vi "CANopenVM_57_single.vi"(0 "node-ID":u8=1 min=1 max=127 step=1, 1 "目标速度":i16=50) -> (2 "电机绝对位置":i32=443333152, 3 "速度反馈值":i32=300, 4 "转矩反馈值 0.1%":i16=40)   [LabVIEW 2020]
uses:
  <vilib>/Platform/TimedLoop/XDataNode/timing_clust.ctl
  <vilib>/Platform/TimedLoop/XDataNode/nitl_modes.ctl
  <vilib>/Platform/TimedLoop/XDataNode/wakeup.ctl
  <vilib>/CANopenLib/CANOPEN.llb/CANopen Interface Create.vi
  <vilib>/CANopenLib/CANOPEN.llb/CANopen SDO Create.vi
  <vilib>/CANopenLib/CANOPEN.llb/CANopen SDO Write [I16].vi
  <vilib>/CANopenLib/CANOPEN.llb/CANopen SDO Close.vi
  <vilib>/CANopenLib/CANOPEN.llb/CANopen SYNC Create.vi
  <vilib>/CANopenLib/CANOPEN.llb/CANopen RPDO Create.vi
  <vilib>/CANopenLib/CANOPEN.llb/CANopen TPDO Create.vi
  <vilib>/CANopenLib/CANOPEN.llb/CANopen TPDO Start.vi
  <vilib>/CANopenLib/CANOPEN.llb/CANopen SYNC Start.vi
  <vilib>/CANopenLib/CANOPEN.llb/CANopen RPDO Start.vi
  <vilib>/CANopenLib/CANOPEN.llb/CANopen Convert To Data [I16].vi
  <vilib>/CANopenLib/CANOPEN.llb/CANopen Fetch from Data [I16].vi
  <vilib>/CANopenLib/CANOPEN.llb/CANopen Fetch from Data [I32].vi
  <vilib>/CANopenLib/CANOPEN.llb/CANopen SYNC Close.vi
  <vilib>/CANopenLib/CANOPEN.llb/CANopen RPDO Close.vi
  <vilib>/CANopenLib/CANOPEN.llb/CANopen TPDO Close.vi
  <vilib>/CANopenLib/CANOPEN.llb/CANopen Interface Close.vi
  <vilib>/Platform/TimedLoop/XDataNode/XDataNode.xnode
  <vilib>/Platform/TimedLoop/XDataNode/XDNodeRunTimeDep.lvlib
panel:
  out "completion code 4":u32
  out "completion code 3":u32
  out "completion code":u32
  in  "buffer size (0) 2":u16
  in  "TPDO channel":u8(ring)=2 items=["PDO 1", "PDO 2", "PDO 3", "PDO 4"]
  in  "Set Target Vilocity":i16
  in  "stop":bool
  out "timestamp":timestamp=timestamp(3824613290.037175 s since 1904-01-01)
  in  "buffer size (0)":u16=10
  in  "TPDO channel read":u8(ring)=1 items=["PDO 1", "PDO 2", "PDO 3", "PDO 4"]
  in  "RPDO channel write":u8(ring)=1 items=["PDO 1", "PDO 2", "PDO 3", "PDO 4"]
  in  "period (ms)":i64=10
  out "completion code 2":u32
  out "completion code 1":u32
  in  "batch SDO name":string="NiMotion_VM"
  in  "baud rate":u32(ring) items=["1 Mbit/s"=0, "800 kbit/s"=1, "500 kbit/s"=2, "250 kbit/s"=3, "125 kbit/s"=4, "50 kbit/s"=6, "20 kbit/s"=7, "10 kbit/s"=8]
  in  "CANopen interface":u32(ring) items=["CANopen01", "CANopen02", "CANopen03", "CANopen04", "CANopen05", "CANopen06", "CANopen07", "CANopen08", "CANopen09", "CANopen10", "CANopen11", "CANopen12", "CANopen13", "CANopen14", "CANopen15", "CANopen16", "CANopen17", "CANopen18", "CANopen19", "CANopen20", "CANopen21", "CANopen22", "CANopen23", "CANopen24", "CANopen25", "CANopen26", "CANopen27", "CANopen28", "CANopen29", "CANopen30", "CANopen31", "CANopen32"]
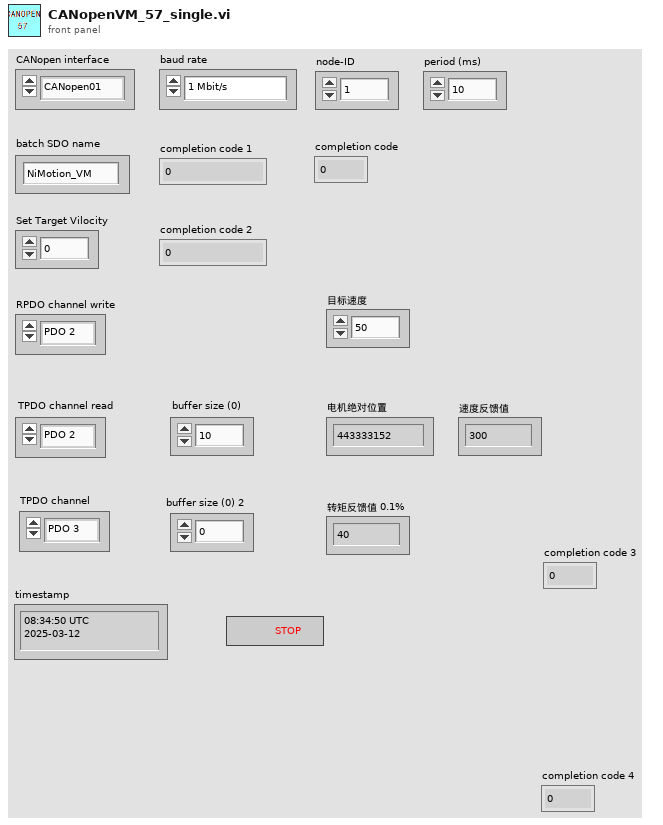
[diagram p1: front panel]
types:
  T1 = typedef "XDNodeRunTimeDep.lvlib/timing_clust.ctl" = cluster{"Expected End [f-1]":u64, "Actual End [f-1]":u64, "Finished Late? [f-1]":bool, "Expected End [i-1]":u64, "Actual End [i-1]":u64, "Finished Late? [i-1]":bool, "Expected Start [i]":u64, "Actual Start [i]":u64, "Expected Start [f]":u64, "Actual Start [f]":u64, "Source Name":string, "Structure Name":string, "Period":i64, "Deadline":i64, "Offset":i64, "Start":i64, "Priority":i32, "Timeout":i32, "Mode":T2, "Wakeup Reason":T3, "Error":errorcluster, "Source Type":string, "Secondary Source Type":string, "Global End Time":u64, "Global Start Time":u64, "Frame Duration":u64, "Iteration Duration":u64, "Assigned CPU":i32, "I/O Scan Engine Mode":u32}
  T2 = typedef "XDNodeRunTimeDep.lvlib/nitl_modes.ctl" = enum32{"No Change", "Process missed periods, maintain original phase", "Discard missed periods, maintain original phase", "Process missed periods, ignore original phase", "Discard missed periods, ignore original phase"}
  T3 = typedef "XDNodeRunTimeDep.lvlib/wakeup.ctl" = enum32{"Normal", "Aborted", "Asynchronous wakeup", "Timing source error", "Timed loop error", "Timeout"}
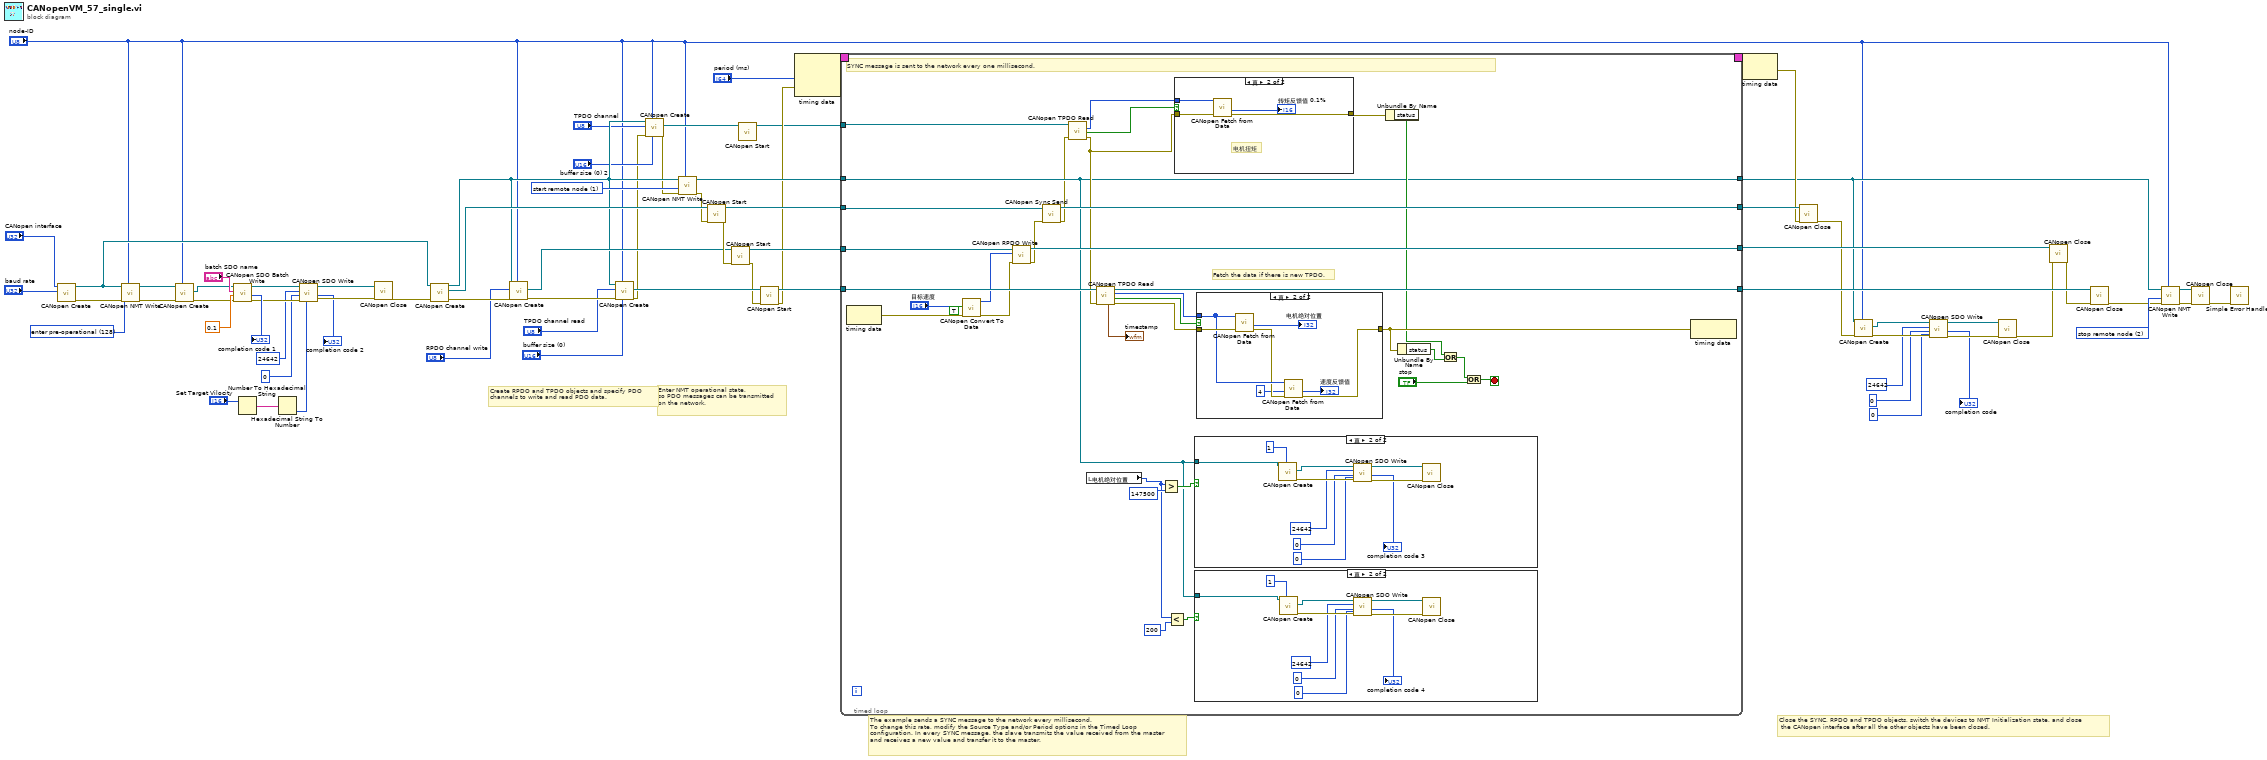
[diagram p0: block diagram]
diagram:
  w37 = u16 2 items=["start remote node"=1, "stop remote node"=2, "enter pre-operational"=128, "reset node"=129, "reset communication"=130] ("command")
  w49 = u16 1 items=["start remote node"=1, "stop remote node"=2, "enter pre-operational"=128, "reset node"=129, "reset communication"=130] ("command")
  w65 = u16 128 items=["start remote node"=1, "stop remote node"=2, "enter pre-operational"=128, "reset node"=129, "reset communication"=130] ("command")
  # "SYNC message is sent to the network every one millisecond."
  # "Close the SYNC, RPDO and TPDO objects, switch the devices to NMT Initialization state, and close\n the CANopen interface after all the other objects have been closed."
  # "The example sends a SYNC message to the network every millisecond.\nTo change this rate, modify the Source Type and/or Period options in the Timed Loop\nconfiguration. In every SYNC message, the slave transmits the value received from the master\nand receives a new value and transfer it to the master."
  # "Enter NMT operational state,\nso PDO messages can be transmitted\non the network."
  # "Create RPDO and TPDO objects and specify PDO \nchannels to write and read PDO data."
  n1 = call-poly <vilib>:"CANopen Create.vi"("baud rate"="baud rate", "interface name"="CANopen interface") -> ("error out"=w66:errorcluster, "interface object out"=w41:refnum<k20>)  [unwired: 8 in]
  n2 = call <vilib>:"CANopen NMT Write.vi"("node-ID (0)"="node-ID", "error in (no error)"=w66, "command"=w65, "interface object in"=w41) -> ("error out"=w69:errorcluster, "interface object out"=w70:refnum<k20>)  [unwired: 6 in]
  n3 = call-poly <vilib>:"CANopen Create.vi"("node-ID"="node-ID", "error in (no error)"=w69, "interface object in"=w70) -> ("error out"=w56:errorcluster, "SDO object out"=w62:refnum<k20>)  [unwired: 6 in, 1 out]
  n4 = call <vilib>:"CANopen SDO Batch Write.vi"("error in (no error)"=w56, "timeout (1s)"=0.1 ("timeout (0s)"), "batch SDO name"="batch SDO name", "SDO object in"=w62) -> ("error out"=w57:errorcluster, "completion code"=→"completion code 1":u32, "SDO object out"=w60:refnum<k20>)  [unwired: 5 in]
  n5 = Number To Hexadecimal String(2:"Set Target Vilocity") -> (0:w24:string)  [unwired: 1 in]
  n6 = Hexadecimal String To Number(string=w24) -> (number=w22:u32)  [unwired: 2 in, 1 out]
  n7 = call-poly <vilib>:"CANopen SDO Write.vi"("I16 data"=w22, "error in (no error)"=w57, "object sub-index (0)"=u8 0, "object index"=u16 24642, "SDO object in"=w60) -> ("error out"=w58:errorcluster, "completion code"=→"completion code 2":u32, "SDO object out"=w59:refnum<k20>)  [unwired: 4 in]
  n8 = call-poly <vilib>:"CANopen Close.vi"("error in (no error)"=w58, "SDO object in"=w59) -> ("error out"=w40:errorcluster)  [unwired: 9 in]
  n9 = call-poly <vilib>:"CANopen Create.vi"("error in (no error)"=w40, "interface object in"=w41) -> ("error out"=w51:errorcluster, "SYNC object out"=w50:refnum<k20>, "interface object out"=w20:refnum<k20>)  [unwired: 7 in]
  n10 = call-poly <vilib>:"CANopen Create.vi"("node-ID"="node-ID", "error in (no error)"=w51, "PDO channel"="RPDO channel write", "interface object in"=w20) -> ("error out"=w45:errorcluster, "RPDO object out"=w44:refnum<k20>)  [unwired: 5 in, 1 out]
  n11 = call-poly <vilib>:"CANopen Create.vi"("buffer size (0)"="buffer size (0)", "node-ID"="node-ID", "error in (no error)"=w45, "PDO channel"="TPDO channel read", "interface object in"=w20) -> ("error out"=w15:errorcluster, "TPDO object out"=w53:refnum<k20>)  [unwired: 4 in, 1 out]
  n12 = call-poly <vilib>:"CANopen Create.vi"("buffer size (0)"="buffer size (0) 2", "node-ID"="node-ID", "error in (no error)"=w15, "PDO channel"="TPDO channel", "interface object in"=w20) -> ("error out"=w14:errorcluster, "TPDO object out"=w17:refnum<k20>)  [unwired: 4 in, 1 out]
  n13 = call <vilib>:"CANopen NMT Write.vi"("node-ID (0)"="node-ID", "error in (no error)"=w14, "command"=w49, "interface object in"=w20) -> ("error out"=w48:errorcluster, "interface object out"=w29:refnum<k20>)  [unwired: 6 in]
  n14 = call-poly <vilib>:"CANopen Start.vi"("error in (no error)"=w48, "SYNC object in"=w50) -> ("error out"=w47:errorcluster, "SYNC object out"=w28:refnum<k20>)  [unwired: 8 in]
  n15 = call-poly <vilib>:"CANopen Start.vi"("error in (no error)"=w47, "RPDO object in"=w44) -> ("error out"=w46:errorcluster, "RPDO object out"=w27:refnum<k20>)  [unwired: 8 in]
  n16 = call-poly <vilib>:"CANopen Start.vi"("TPDO object in"=w17) -> ("TPDO object out"=w16:refnum<k20>)  [unwired: 9 in, 1 out]
  n17 = call-poly <vilib>:"CANopen Start.vi"("error in (no error)"=w46, "TPDO object in"=w53) -> ("error out"=w25:errorcluster, "TPDO object out"=w26:refnum<k20>)  [unwired: 8 in]
  n18 = node-c288("period (ms)", w25) -> (w72:T1)  [unwired: 1 in]
  n19 = timed-loop {
    timing: w72 -> [_]
    timing-out: [_] -> w71
    tunnel: w28 -> [w106]
    tunnel: [w97] -> w33
    tunnel: [w75] -> w12
    tunnel: w29 -> [w75]
    tunnel: w27 -> [w100]
    tunnel: w26 -> [w101]
    tunnel: [w99] -> w36
    tunnel: [w98] -> w13
    tunnel: w16 -> [w89]
    stop <- w105 stop-if-true
    # "Fetch the data if there is new TPDO."
    n20 = node-c288() -> (w91:errorcluster)  [unwired: 1 in]
    n21 = call-poly <vilib>:"CANopen Convert To Data.vi"("trim"=TRUE, "error in (no error)"=w91, "signed 16-bit integer"="目标速度") -> ("error out"=w81:errorcluster, "CANopen data out"=w90:u8[])  [unwired: 7 in]
    n22 = call <vilib>:"CANopen RPDO Write.vi"("error in (no error)"=w81, "data"=w90, "RPDO object in"=w100) -> ("error out"=w74:errorcluster, "RPDO object out"=w98:refnum<k20>)  [unwired: 7 in]
    n23 = call <vilib>:"CANopen Sync Send.vi"("error in (no error)"=w74, "SYNC object in"=w106) -> ("error out"=w73:errorcluster, "SYNC object out"=w97:refnum<k20>)  [unwired: 8 in]
    n24 = call <vilib>:"CANopen TPDO Read.vi"("error in (no error)"=w73, "TPDO object in"=w89) -> ("error out"=w86:errorcluster, "new data?"=w87:bool, "data"=w88:u8[])  [unwired: 5 in, 2 out]
    n25 = local read "电机绝对位置"() -> (w77:i32)
    n26 = call <vilib>:"CANopen TPDO Read.vi"("error in (no error)"=w86, "TPDO object in"=w101) -> ("error out"=w102:errorcluster, "new data?"=w96:bool, "data"=w94:u8[], "TPDO object out"=w99:refnum<k20>, "timestamp"=→"timestamp":timestamp)  [unwired: 5 in]
    n27 = Greater?(x=w77, y=147500) -> (0:w80:bool)
    n28 = Less?(x=w77, y=200) -> (x < y?=w78:bool)
    n29 = case shown="真" w87 {
      tunnel: w86 -> [w127 w131]
      tunnel: w88 -> [_ w130]
      tunnel: [w127 w129] -> w85
      frame False {
      }
      frame True {
        # "电机扭矩"
        n30 = call-poly <vilib>:"CANopen Fetch from Data.vi"("error in (no error)"=w131, "CANopen data in"=w130) -> ("error out"=w129:errorcluster, "signed 16-bit integer"=→"转矩反馈值 0.1%":i16)  [unwired: 7 in, 1 out]
      }
    }
    n31 = case shown="真" w80 {
      tunnel: w75 -> [_ w117]
      frame False {
      }
      frame True {
        n32 = call-poly <vilib>:"CANopen Create.vi"("node-ID"=u8 1, "interface object in"=w117) -> ("error out"=w124:errorcluster, "SDO object out"=w126:refnum<k20>)  [unwired: 7 in, 1 out]
        n33 = call-poly <vilib>:"CANopen SDO Write.vi"("I16 data"=i16 0, "error in (no error)"=w124, "object sub-index (0)"=u8 0 ("sub-index"), "object index"=u16 24642, "SDO object in"=w126) -> ("error out"=w123:errorcluster, "completion code"=→"completion code 3":u32, "SDO object out"=w125:refnum<k20>)  [unwired: 4 in]
        n34 = call-poly <vilib>:"CANopen Close.vi"("error in (no error)"=w123, "SDO object in"=w125) -> ()  [unwired: 9 in, 1 out]
      }
    }
    n35 = case shown="真" w78 {
      tunnel: w75 -> [_ w107]
      frame False {
      }
      frame True {
        n36 = call-poly <vilib>:"CANopen Create.vi"("node-ID"=u8 1, "interface object in"=w107) -> ("error out"=w114:errorcluster, "SDO object out"=w116:refnum<k20>)  [unwired: 7 in, 1 out]
        n37 = call-poly <vilib>:"CANopen SDO Write.vi"("I16 data"=i16 0, "error in (no error)"=w114, "object sub-index (0)"=u8 0 ("sub-index"), "object index"=u16 24642, "SDO object in"=w116) -> ("error out"=w113:errorcluster, "completion code"=→"completion code 4":u32, "SDO object out"=w115:refnum<k20>)  [unwired: 4 in]
        n38 = call-poly <vilib>:"CANopen Close.vi"("error in (no error)"=w113, "SDO object in"=w115) -> ()  [unwired: 9 in, 1 out]
      }
    }
    n39 = case shown="真" w96 {
      tunnel: w102 -> [w137 w144]
      tunnel: w94 -> [_ w143]
      tunnel: [w137 w141] -> w95
      frame False {
      }
      frame True {
        n40 = call-poly <vilib>:"CANopen Fetch from Data.vi"("error in (no error)"=w144, "CANopen data in"=w143) -> ("error out"=w142:errorcluster, "signed 32-bit integer"=→"电机绝对位置":i32)  [unwired: 7 in, 1 out]
        n41 = call-poly <vilib>:"CANopen Fetch from Data.vi"("error in (no error)"=w142, "offset (0)"=u32 4, "CANopen data in"=w143) -> ("error out"=w141:errorcluster, "signed 32-bit integer"=→"速度反馈值":i32)  [unwired: 6 in, 1 out]
      }
    }
    n42 = Unbundle By Name(w85) -> ("status"=w83:bool)
    n43 = Unbundle By Name(w95) -> ("status"=w84:bool)
    n44 = Or(x=w83, y=w84) -> (x .or. y?=w82:bool)
    n45 = Or(x=w82, y="stop") -> (x .or. y?=w105:bool)
    n46 = node-c288(w95) -> ()  [unwired: 1 out]
  }
  n47 = node-c288(w71) -> (w31:errorcluster)
  n48 = call-poly <vilib>:"CANopen Close.vi"("error in (no error)"=w31, "SYNC object in"=w33) -> ("error out"=w9:errorcluster)  [unwired: 9 in]
  n49 = call-poly <vilib>:"CANopen Create.vi"("node-ID"="node-ID", "error in (no error)"=w9, "interface object in"=w12) -> ("error out"=w8:errorcluster, "SDO object out"=w11:refnum<k20>)  [unwired: 6 in, 1 out]
  n50 = call-poly <vilib>:"CANopen SDO Write.vi"("I16 data"=i16 0, "error in (no error)"=w8, "object sub-index (0)"=u8 0 ("sub-index"), "object index"=u16 24642, "SDO object in"=w11) -> ("error out"=w7:errorcluster, "completion code"=→"completion code":u32, "SDO object out"=w10:refnum<k20>)  [unwired: 4 in]
  n51 = call-poly <vilib>:"CANopen Close.vi"("error in (no error)"=w7, "SDO object in"=w10) -> ("error out"=w6:errorcluster)  [unwired: 9 in]
  n52 = call-poly <vilib>:"CANopen Close.vi"("error in (no error)"=w6, "RPDO object in"=w13) -> ("error out"=w35:errorcluster)  [unwired: 9 in]
  n53 = call-poly <vilib>:"CANopen Close.vi"("error in (no error)"=w35, "TPDO object in"=w36) -> ("error out"=w34:errorcluster)  [unwired: 9 in]
  n54 = call <vilib>:"CANopen NMT Write.vi"("node-ID (0)"="node-ID", "error in (no error)"=w34, "command"=w37, "interface object in"=w12) -> ("error out"=w39:errorcluster, "interface object out"=w38:refnum<k20>)  [unwired: 6 in]
  n55 = call-poly <vilib>:"CANopen Close.vi"("error in (no error)"=w39, "interface object in"=w38) -> ("error out"=w32:errorcluster)  [unwired: 9 in]
  n56 = call <vilib>:"Simple Error Handler.vi"("error in (no error)"=w32) -> ()  [unwired: 4 in, 5 out]
